vi "dkin.vi"(8 "phi_r":dbl min=-12.5664 max=12.5664 step=0.01, 11 "phi_d":dbl min=-12.5664 max=12.5664 step=0.01) -> (0 "w":dbl, 3 "v":dbl)   [LabVIEW 2019]
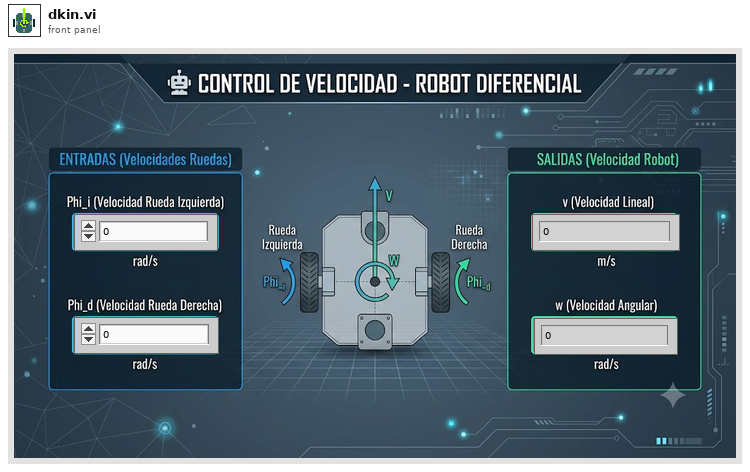
[diagram p1: front panel]
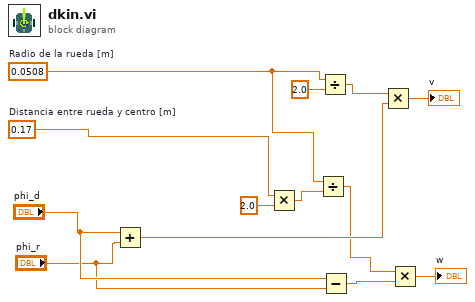
[diagram p0: block diagram]
diagram:
  w7 = 0.17  # Distancia entre rueda y centro [m]
  w6 = 0.0508  # Radio de la rueda [m]
  n1 = Add(x="phi_d", y="phi_r") -> (x+y=w11:dbl)
  n2 = Multiply(x=w7, y=2.0) -> (x*y=w9:dbl)
  n3 = Divide(x=w6, y=w9) -> (x/y=w4:dbl)
  n4 = Divide(x=w6, y=2.0) -> (x/y=w12:dbl)
  n5 = Subtract(x="phi_d", y="phi_r") -> (x-y=w3:dbl)
  n6 = Multiply(x=w12, y=w11) -> (x*y=→"v":dbl)
  n7 = Multiply(x=w4, y=w3) -> (x*y=→"w":dbl)
